vi "Door_backup.vi"(0 "Strings in":string[](array[string])=["C:\\CuspControl\\GPIB and Network\\Cusp\\Dummyfile.txt", "6723"], 1 "Dubs in":dbl[](array[numeric])=[0.0]) -> ()   [LabVIEW 2018]
uses:
  <vilib>/Analysis/1siggen.llb/Ramp Pattern by Samples.vi
  <vilib>/DAQmx/write.llb/DAQmx Write (Analog DBL 1Chan 1Samp).vi
  <vilib>/DAQmx/create/channels.llb/DAQmx Create Channel (AO-Voltage-Basic).vi
  <vilib>/DAQmx/miscellaneous.llb/DAQmx Fill In Error Info.vi
  <vilib>/Analysis/NI_AALBase.lvlib
panel:
  out "Ramp Pattern":dbl[](array[numeric])
  in  "samples":i32=128
  in  "file (use dialog)":path=path "C:/CuspControl/GPIB and Network/Cusp/DoorVolts.txt"
  in  "subvi":bool=TRUE
  out "error out":errorcluster
  in  "AO2 name":string="6723"
  in  "Takasago Vc ao line":string="/ao12"
  in  "ON voltage":dbl format="%#_13g"
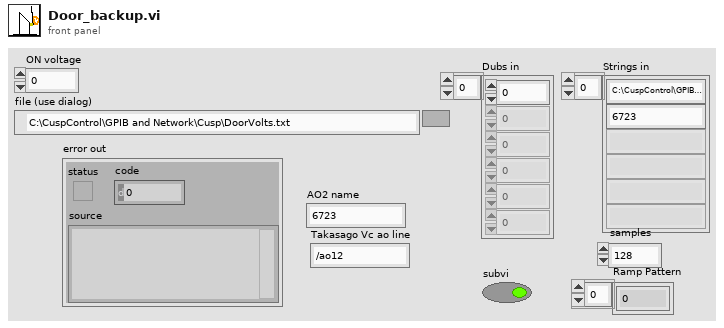
[diagram p1: front panel]
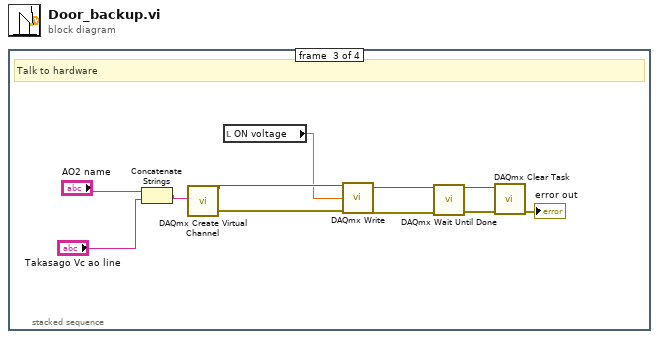
[diagram p0: block diagram]
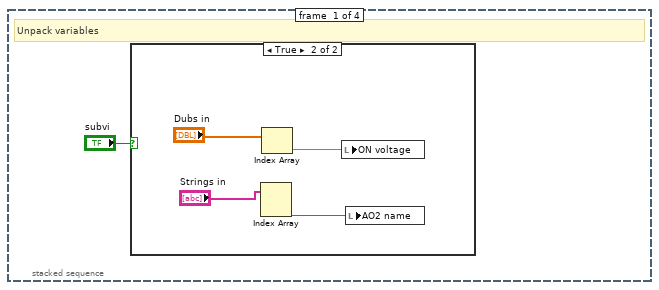
[diagram p2: hidden frame]
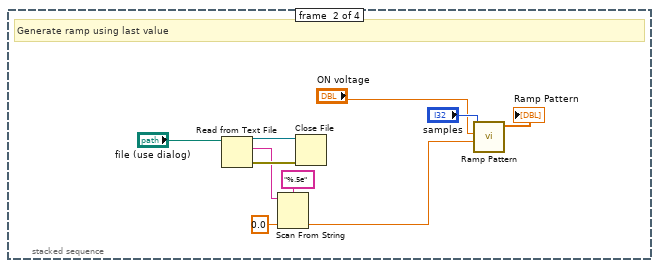
[diagram p4: hidden frame]
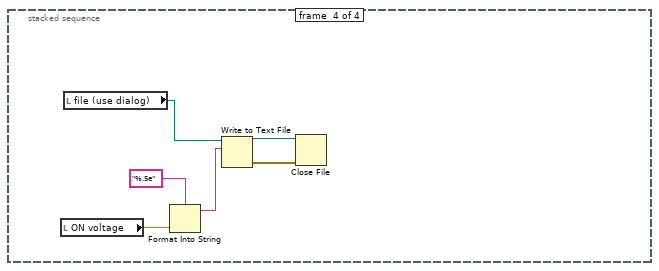
[diagram p5: hidden frame]
diagram:
  n1 = stacked-sequence {
    frame #0 {
      # "Unpack variables"
      n2 = case shown="True" "subvi" {
        frame False {
        }
        frame True {
          n3 = Index Array(array="Strings in") -> (element #2=w2:string)  [unwired: 2 in, 1 out]
          n4 = Index Array(array="Dubs in") -> (element=w3:dbl)  [unwired: 1 in]
          n5 = local write "ON voltage"(w3) -> ()
          n6 = local write "AO2 name"(w2) -> ()
        }
      }
    }
    frame #1 {
      # "Generate ramp using last value"
      n7 = Read from Text File(file (use dialog)="file (use dialog)") -> (refnum out=w14:refnum<file>, text=w12:string, error out=w13:errorcluster)  [unwired: 3 in, 1 out]
      n8 = Scan From String(format string="%.5e", input string=w12, default 1=0.0 ("default value 1")) -> (output 1=w9:dbl)  [unwired: 2 in, 3 out]
      n9 = Close File(refnum=w14, error in=w13) -> ()  [unwired: 2 out]
      n10 = call-poly <vilib>:"Ramp Pattern.vi"("start"=w9, "end"="ON voltage", "samples"="samples") -> ("Ramp Pattern"=→"Ramp Pattern":dbl[])  [unwired: 7 in, 1 out]
    }
    frame #2 {
      # "Talk to hardware"
      n11 = Concatenate Strings("AO2 name", "Takasago Vc ao line") -> (w22:string)
      n12 = call-poly <vilib>:"DAQmx Create Virtual Channel.vi"("physical channels"=w22) -> ("task out"=w18:refnum<k21>, "error out"=w17:errorcluster)  [unwired: 13 in]
      n13 = local read "ON voltage"() -> (w16:dbl)
      n14 = call-poly <vilib>:"DAQmx Write.vi"("task/channels in"=w18, "data"=w16, "error in"=w17) -> ("task out"=w24:refnum<k21>, "error out"=w23:errorcluster)  [unwired: 10 in, 1 out]
      n15 = call <vilib>:"DAQmx Wait Until Done.vi"("task/channels in"=w24, "error in"=w23) -> ("task out"=w26:refnum<k21>, "error out"=w25:errorcluster)  [unwired: 12 in]
      n16 = call <vilib>:"DAQmx Clear Task.vi"("task in"=w26, "error in"=w25) -> ("error out"=→"error out":errorcluster)  [unwired: 13 in]
    }
    frame #3 {
      n17 = local read "ON voltage"() -> (w29:dbl)
      n18 = local read "file (use dialog)"() -> (w30:path)
      n19 = Format Into String(format string="%.5e", w29) -> (resulting string=w28:string)  [unwired: 2 in, 1 out]
      n20 = Write to Text File(file (use dialog)=w30, text=w28) -> (refnum out=w32:refnum<file>, error out=w31:errorcluster)  [unwired: 2 in, 1 out]
      n21 = Close File(refnum=w32, error in=w31) -> ()  [unwired: 2 out]
    }
  }
